vi "Pre Launch Init.vi"(11 "Actor_NI6008 in":refnum<class "Actor_NI6008.lvclass">) -> (0 "error out":errorcluster, 3 "Actor_NI6008 out":refnum<class "Actor_NI6008.lvclass">)   [LabVIEW 2020, in "Actor_NI6008.lvlib" / "Actor_NI6008.lvclass"]
doc: "(<B>Filename</B>: Actor Framework.lvlib:Actor.lvclass:Pre Launch Init.vi)\n\nDefines behavior that occurs after the Launch Nested Actor method is invoked but before the actor's Actor Core method begins running.\n\nBy default, this method does nothing. A descendant class may override it to define behavior."
uses:
  Actor_NI6008.lvclass
  C:/Program Files/National Instruments/LabVIEW 2020/vi.lib/ActorFramework/Actor/Actor.lvclass
  Actor_NI6008.lvclass/Actor_NI6008.ctl
  <vilib>/ActorFramework/Actor/Actor.lvclass/Actor.ctl
  I_NI6008 Messages/NI6008 Status Report Msg/NI6008 Status Report Msg.lvclass/NI6008 Status Report Msg.ctl
  <vilib>/ActorFramework/Message Enqueuer/Message Enqueuer.lvclass/Message Enqueuer.ctl
  <vilib>/DAQmx/write.llb/DAQmx Write (Digital 1D Bool NChan 1Samp 1Line).vi
  <vilib>/DAQmx/write.llb/DAQmx Write (Digital Bool 1Line 1Point).vi
  <vilib>/DAQmx/read.llb/DAQmx Read (Analog DBL 1Chan 1Samp).vi
  <vilib>/ActorFramework/Message Enqueuer/Enqueue.vi
  I_NI6008 Messages/NI6008 Status Report Msg/NI6008 Status Report Msg.lvclass
  C:/Program Files/National Instruments/LabVIEW 2020/vi.lib/ActorFramework/Message/Message.lvclass
  <vilib>/DAQmx/create/channels.llb/DAQmx Create Channel (DO-Digital Output).vi
  <vilib>/DAQmx/miscellaneous.llb/DAQmx Fill In Error Info.vi
  <vilib>/DAQmx/create/channels.llb/DAQmx Create Channel (AI-Voltage-Basic).vi
  <vilib>/ActorFramework/Message Priority Queue/Priority Enqueue.vi
  <vilib>/ActorFramework/Actor/Actor.lvclass
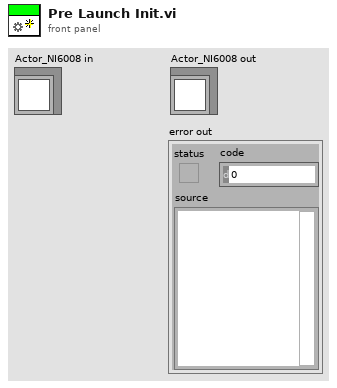
[diagram p1: front panel]
types:
  T1 = cluster{"Msg":string, "DO":bool[], "AI":dbl, "NI6008 Error":errorcluster}
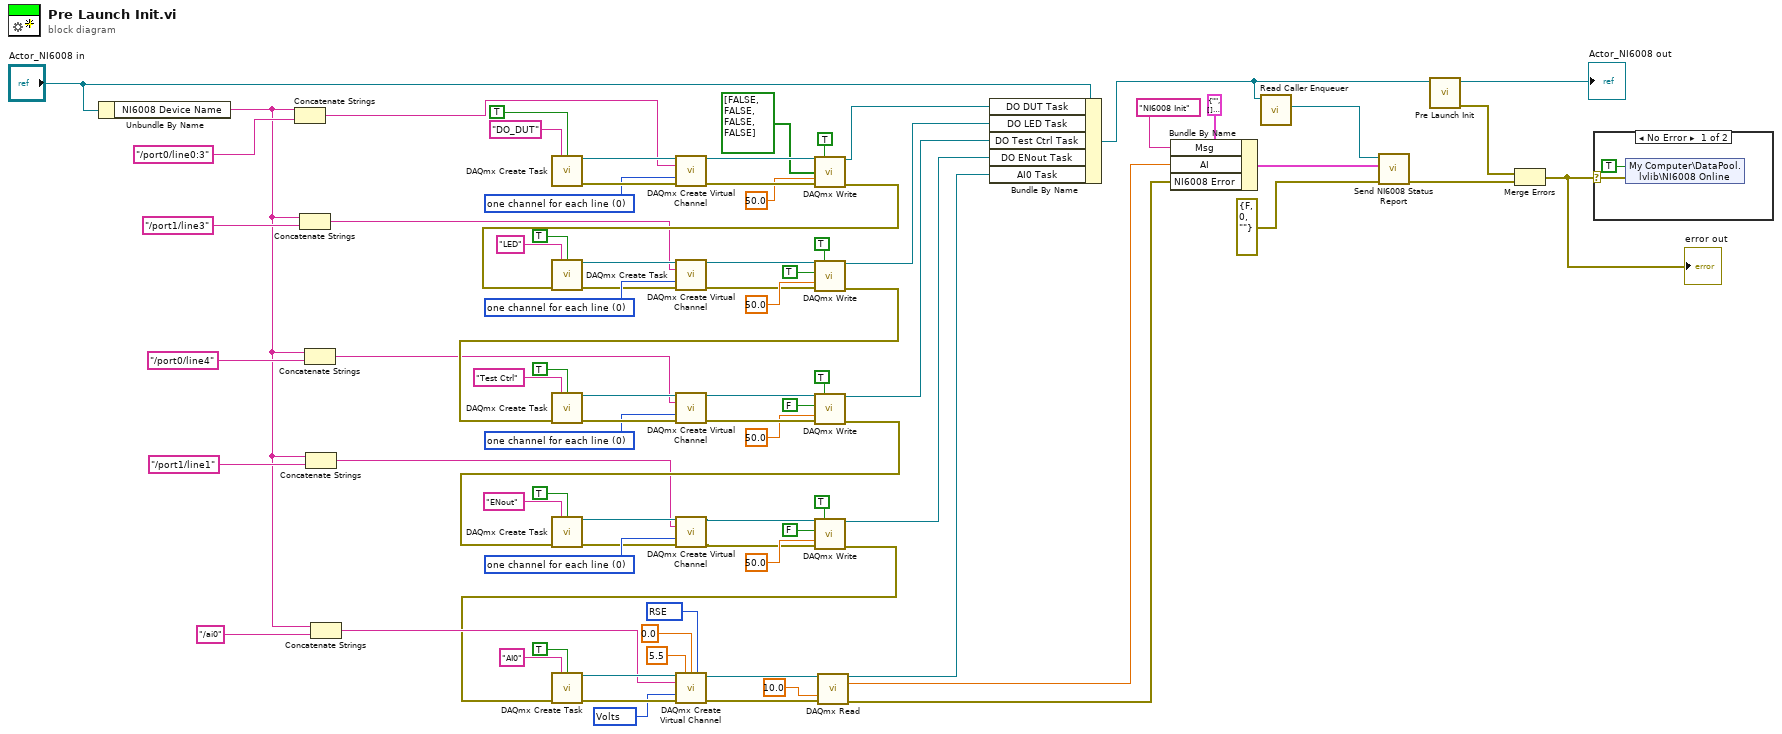
[diagram p0: block diagram]
diagram:
  w32 = 10348 items=["Volts"=10348, "From Custom Scale"=10065] ("units")
  w33 = 10083 items=["Default"=-1, "RSE"=10083, "NRSE"=10078, "Differential"=10106, "Pseudodifferential"=12529] ("input terminal configuration")
  w45 = 0 items=["one channel for each line", "one channel for all lines"] ("line grouping")
  w49 = 0 items=["one channel for each line", "one channel for all lines"] ("line grouping")
  w60 = 0 items=["one channel for each line", "one channel for all lines"] ("line grouping")
  w79 = 0 items=["one channel for each line", "one channel for all lines"] ("line grouping")
  n1 = Unbundle By Name("Actor_NI6008 in") -> ("NI6008 Device Name"=w13:tag)
  n2 = Concatenate Strings(w13, "/port0/line0:3" ("string")) -> (w12:string)
  n3 = Concatenate Strings(w13, "/port1/line3" ("string")) -> (w11:string)
  n4 = Concatenate Strings(w13, "/port0/line4" ("string")) -> (w10:string)
  n5 = Concatenate Strings(w13, "/port1/line1" ("string")) -> (w9:string)
  n6 = Concatenate Strings(w13, "/ai0" ("string")) -> (w8:string)
  n7 = call <vilib>:"DAQmx Create Task.vi"("new task name"="DO_DUT", "auto cleanup"=TRUE) -> ("task out"=w81:refnum<k21>, "error out"=w80:errorcluster)  [unwired: 12 in]
  n8 = call-poly <vilib>:"DAQmx Create Virtual Channel.vi"("task in"=w81, "lines"=w12, "line grouping"=w79, "error in"=w80) -> ("task out"=w78:refnum<k21>, "error out"=w77:errorcluster)  [unwired: 10 in]
  n9 = call-poly <vilib>:"DAQmx Write.vi"("task/channels in"=w78, "auto start"=TRUE, "data"=bool[] [FALSE, FALSE, FALSE, FALSE], "timeout"=50.0, "error in"=w77) -> ("task out"=w66:refnum<k21>, "error out"=w41:errorcluster)  [unwired: 8 in, 1 out]
  n10 = call <vilib>:"DAQmx Create Task.vi"("new task name"="LED", "auto cleanup"=TRUE, "error in"=w41) -> ("task out"=w58:refnum<k21>, "error out"=w59:errorcluster)  [unwired: 11 in]
  n11 = call-poly <vilib>:"DAQmx Create Virtual Channel.vi"("task in"=w58, "lines"=w11, "line grouping"=w60, "error in"=w59) -> ("task out"=w61:refnum<k21>, "error out"=w62:errorcluster)  [unwired: 10 in]
  n12 = call-poly <vilib>:"DAQmx Write.vi"("task/channels in"=w61, "auto start"=TRUE, "data"=TRUE, "timeout"=50.0, "error in"=w62) -> ("task out"=w28:refnum<k21>, "error out"=w40:errorcluster)  [unwired: 8 in, 1 out]
  n13 = call <vilib>:"DAQmx Create Task.vi"("new task name"="Test Ctrl", "auto cleanup"=TRUE, "error in"=w40) -> ("task out"=w51:refnum<k21>, "error out"=w50:errorcluster)  [unwired: 11 in]
  n14 = call-poly <vilib>:"DAQmx Create Virtual Channel.vi"("task in"=w51, "lines"=w10, "line grouping"=w49, "error in"=w50) -> ("task out"=w48:refnum<k21>, "error out"=w47:errorcluster)  [unwired: 10 in]
  n15 = call-poly <vilib>:"DAQmx Write.vi"("task/channels in"=w48, "auto start"=TRUE, "data"=FALSE, "timeout"=50.0, "error in"=w47) -> ("task out"=w27:refnum<k21>, "error out"=w39:errorcluster)  [unwired: 8 in, 1 out]
  n16 = call <vilib>:"DAQmx Create Task.vi"("new task name"="ENout", "auto cleanup"=TRUE, "error in"=w39) -> ("task out"=w43:refnum<k21>, "error out"=w44:errorcluster)  [unwired: 11 in]
  n17 = call-poly <vilib>:"DAQmx Create Virtual Channel.vi"("task in"=w43, "lines"=w9, "line grouping"=w45, "error in"=w44) -> ("task out"=w4:refnum<k21>, "error out"=w3:errorcluster)  [unwired: 10 in]
  n18 = call-poly <vilib>:"DAQmx Write.vi"("task/channels in"=w4, "auto start"=TRUE, "data"=FALSE, "timeout"=50.0, "error in"=w3) -> ("task out"=w2:refnum<k21>, "error out"=w1:errorcluster)  [unwired: 8 in, 1 out]
  n19 = call <vilib>:"DAQmx Create Task.vi"("new task name"="AI0", "auto cleanup"=TRUE, "error in"=w1) -> ("task out"=w37:refnum<k21>, "error out"=w36:errorcluster)  [unwired: 11 in]
  n20 = call-poly <vilib>:"DAQmx Create Virtual Channel.vi"("task in"=w37, "maximum value"=5.5, "minimum value"=0.0, "input terminal configuration"=w33, "physical channels"=w8, "units"=w32, "error in"=w36) -> ("task out"=w31:refnum<k21>, "error out"=w30:errorcluster)  [unwired: 7 in]
  n21 = call-poly <vilib>:"DAQmx Read.vi"("task/channels in"=w31, "timeout"=10.0, "error in"=w30) -> ("task out"=w26:refnum<k21>, "data"=w25:dbl, "error out"=w24:errorcluster)  [unwired: 10 in]
  n22 = Bundle By Name(cluster="Actor_NI6008 in", "DO DUT Task"=w66, "DO LED Task"=w28, "DO Test Ctrl Task"=w27, "DO ENout Task"=w2, "AI0 Task"=w26) -> (w65:refnum<class "Actor_NI6008.lvclass">)
  n23 = Bundle By Name(cluster=T1 {"Msg"="", "DO"=[], "AI"=0.0, "NI6008 Error"={"status"=FALSE, "code"=0, "source"=""}} ("Data"), "Msg"="NI6008 Init", "AI"=w25, "NI6008 Error"=w24) -> (w71:T1)
  n24 = call <vilib>:"Read Caller Enqueuer.vi"("Actor"=w65) -> ("Caller Enqueuer"=w69:refnum<class "Message Enqueuer.lvclass">)  [unwired: 10 in]
  n25 = call "Send NI6008 Status Report.vi"("error in (no error)"=errorcluster {"status"=FALSE, "code"=0, "source"=""} ("error constant"), "Data"=w71, "Message Enqueuer"=w69) -> ("error out"=w67:errorcluster)  [unwired: 7 in, 1 out]
  n26 = call-parent "Pre Launch Init.vi"("Actor in"=w65) -> ("error out"=w68:errorcluster, "Actor out"=→"Actor_NI6008 out":refnum<class "Actor_NI6008.lvclass">)  [unwired: 9 in]
  n27 = Merge Errors(w68, w67) -> (w64:errorcluster)
  "error out" <- w64
  n28 = case shown="No Error" w64 {
    selector: w64 -> [w86 _]
    frame No Error {
      n29 = shared-variable "My Computer\\DataPool.lvlib\\NI6008 Online"(TRUE ("NI6008 Online"), error in=w86) -> ()  [unwired: 1 out]
    }
    frame Error {
    }
  }
